vi "Close.vi"(8 "error in (no error)":errorcluster, 11 "reference in":refnum<class "PSU_Keysight_34951A.lvclass">) -> (0 "error out":errorcluster, 3 "reference in":refnum<class "PSU_Keysight_34951A.lvclass">)   [LabVIEW 2022 SP3, in "PSU_Keysight_34951A.lvlib" / "PSU_Keysight_34951A.lvclass"]
uses:
  PSU_Keysight_34951A.lvclass
  Components/PSU_Base.lvlibp/PSU_Base.lvclass
  Components/ViPER.lvlibp/ViPER.lvclass
  C:/Projects/Medulla/ViPER/Examples/Flux_Capacitor_Tester/Components/ViPER.lvlibp/ViPER.lvclass
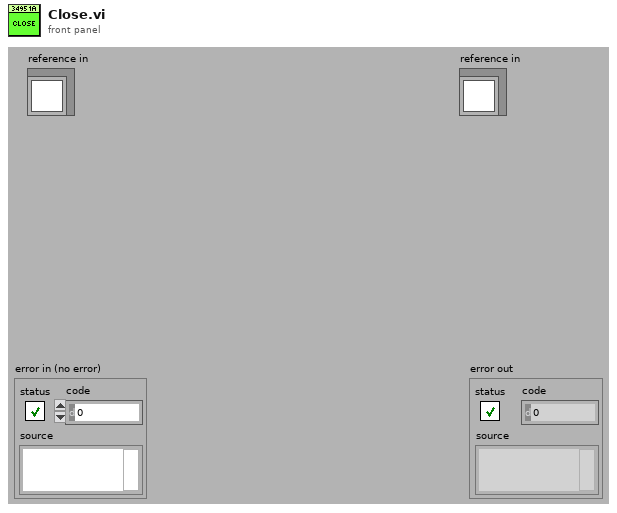
[diagram p1: front panel]
types:
  T1 = typedef "PSU_Keysight_34951A.lvlib/PSU_Keysight_34951A.lvclass/ObjectAttributes.ctl" = cluster{"Config":T2, "VISA res":refnum<visa-resource-name>, "Enabled":bool[], "V":dbl[], "I":dbl[], "Source Type":enum16{"Voltage", "Current"}[]}
  T2 = typedef "PSU_Keysight_34951A.lvlib/PSU_Keysight_34951A.lvclass/Config.ctl" = cluster{"VISA":refnum<visa-resource-name>, "Slot":i32}
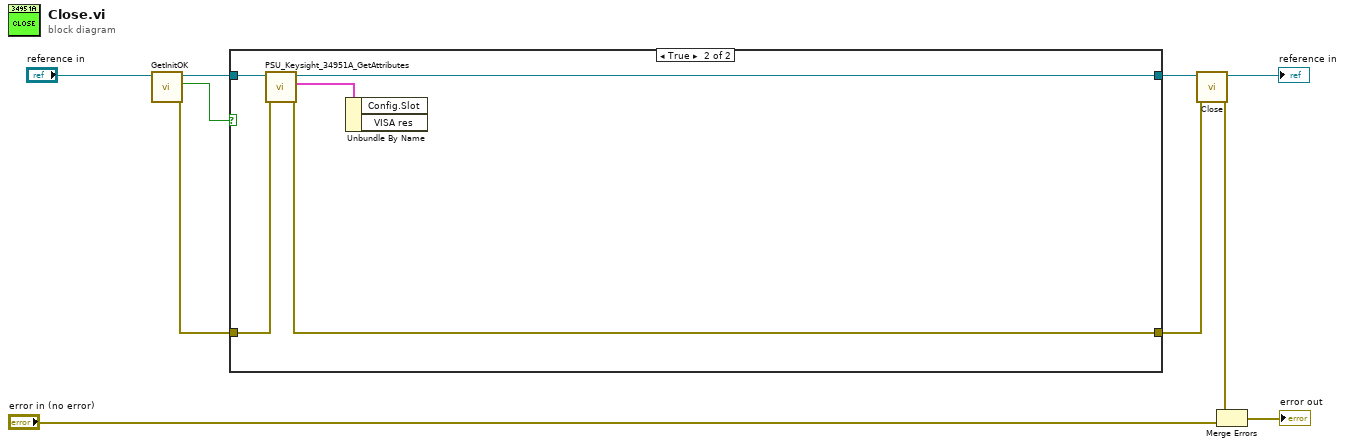
[diagram p0: block diagram]
diagram:
  n1 = call "GetInitOK.vi"("reference in"="reference in") -> ("error out"=w4:errorcluster, "init_ok"=w5:bool, "reference out"=w6:refnum<class "PSU_Keysight_34951A.lvclass">)  [unwired: 8 in]
  n2 = case shown="True" w5 {
    tunnel: w4 -> [w12 w16]
    tunnel: [w12 w13] -> w7
    tunnel: w6 -> [w11 w17]
    tunnel: [w11 w14] -> w8
    frame False {
    }
    frame True {
      n3 = call "PSU_Keysight_34951A_GetAttributes.vi"("error in (no error)"=w16, "reference in"=w17) -> ("error out"=w13:errorcluster, "Data"=w15:T1, "reference out"=w14:refnum<class "PSU_Keysight_34951A.lvclass">)  [unwired: 6 in, 1 out]
      n4 = Unbundle By Name(w15) -> ()  [unwired: 2 out]
    }
  }
  n5 = call-parent "Close.vi"("error in (no error)"=w7, "reference in"=w8) -> ("error out"=w3:errorcluster, "reference in"=→"reference in":refnum<class "PSU_Keysight_34951A.lvclass">)  [unwired: 8 in]
  n6 = Merge Errors(w3, "error in (no error)") -> (→"error out":errorcluster)
